vi "Write lines.vi"(8 "error in":errorcluster, 10 "lines":T1[](array[typedef]), 11 "shared memory module configuration":refnum<class "Shared Memory Configuration.lvclass">) -> (0 "error out":errorcluster, 3 "shared memory module configuration out":refnum<class "Shared Memory Configuration.lvclass">)   [LabVIEW 2013, in "Shared Memory Configuration.lvclass"]
doc: "Copyright 2016 National Instruments Corporation\n\nLicensed under the Apache License, Version 2.0 (the \"License\"); you may not use this file except in compliance with the License. You may obtain a copy of the License at http://www.apache.org/licenses/LICENSE-2.0\nUnless required by applicable law or agreed to in writing, software distributed under the License is distributed on an \"AS IS\" BASIS, WITHOUT WARRANTIES OR CONDITIONS OF ANY KIND, either express or implied. See the License for the specific language governing permissions and limitations under the License."
uses:
  Shared Memory Configuration.lvclass
  line configuration.ctl
  <vilib>/NI/Tag Bus Module Framework/channel/TBM channel.lvclass
  <vilib>/NI/Tag Bus/tag/Data Type.ctl
  Shared Memory Configuration.lvclass/Shared Memory Configuration.ctl
  <vilib>/NI/Tag Bus/tag/tag descriptor.lvclass
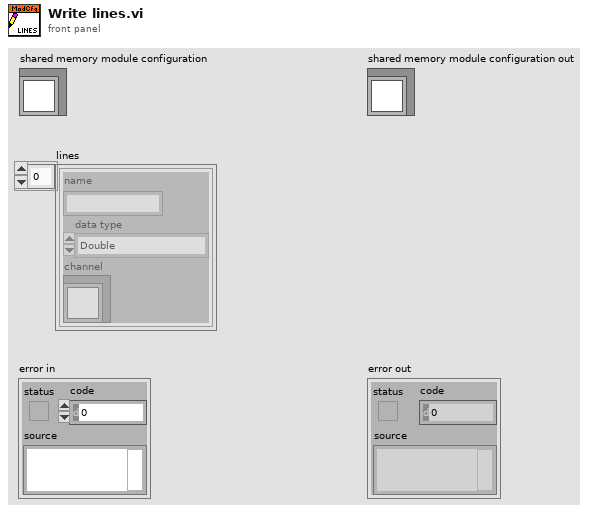
[diagram p1: front panel]
types:
  T1 = typedef "Shared Memory Configuration.lvclass/line configuration.ctl" = cluster{"name":string, "data type":T2, "channel":refnum<class "TBM channel.lvclass">}
  T2 = typedef "tag bus.lvlib/tag descriptor.lvclass/Data Type.ctl" = enum16{"Double", "Single", "I64", "I32", "I16", "I8", "U64", "U32", "U16", "U8", "Boolean", "String", "Array of Double", "Array of Single", "Array of I64", "Array of I32", "Array of I16", "Array of I8", "Array of U64", "Array of U32", "Array of U16", "Array of U8", "Array of Boolean", "Array of String"}
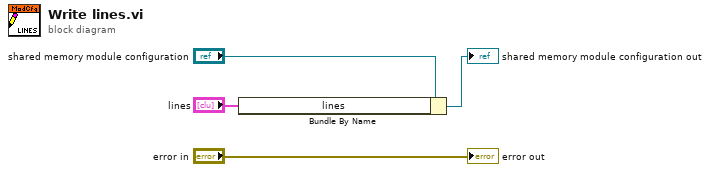
[diagram p0: block diagram]
diagram:
  n1 = Bundle By Name(cluster="shared memory module configuration", "lines"="lines") -> (→"shared memory module configuration out":refnum<class "Shared Memory Configuration.lvclass">)
  "error out" <- "error in"
